vi "PWM_Lenkung.vi"(0 "vorne rechts":dbl=75.31181382488626, 1 "vorne links":dbl=29.917677039556622, 2 "Start":bool, 3 "Schräg links":dbl=31.586166184242515, 4 "Schräg rechts":dbl, 5 "PID Werte":T1={"proportional gain (Kc)"=0.5, "integral time (Ti, min)"=0.0, "derivative time (Td, min)"=0.002} {"proportional gain (Kc)" format="%#_10g"; "integral time (Ti, min)" format="%#_10g"; "derivative time (Td, min)" format="%#_10g"}) -> (14 "PWM Lenkung":dbl=0.3577035044911076)   [LabVIEW 2016]
doc: "PID Regelung für Servowert\n05.04.17_Tloe"
uses:
  <vilib>/addons/control/pid/pid.llb/PID (DBL).vi
  <vilib>/addons/control/pid/NI_PID_pid.lvlib
panel:
  in  "Abweichung (cm)":dbl=20.0 format="%#_13g"
  in  "Anteil Schräg":dbl=0.9
  # "vorher 0,9"
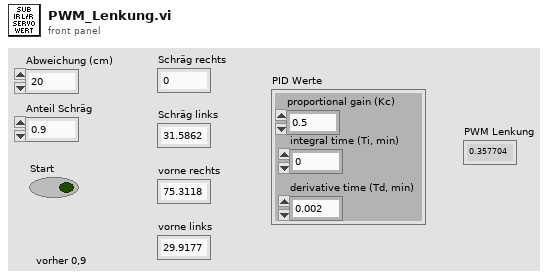
[diagram p1: front panel]
types:
  T1 = cluster{"proportional gain (Kc)":dbl, "integral time (Ti, min)":dbl, "derivative time (Td, min)":dbl}
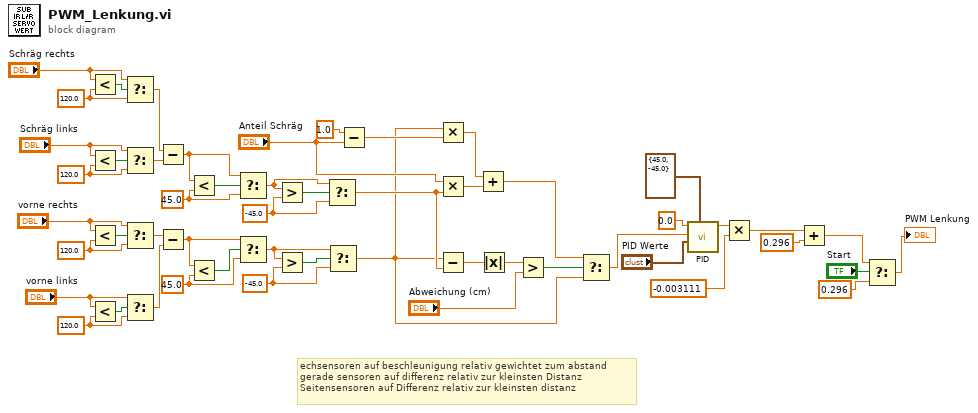
[diagram p0: block diagram]
diagram:
  w22 = 120.0 ("y")
  w26 = 120.0 ("y")
  w30 = 120.0 ("y")
  w33 = 120.0 ("y")
  w36 = -45.0 ("y")
  w39 = 45.0 ("y")
  w41 = -45.0 ("y")
  w44 = 45.0 ("y")
  # "echsensoren auf beschleunigung relativ gewichtet zum abstand\ngerade sensoren auf differenz relativ zur kleinsten Distanz\nSeitensensoren auf Differenz relativ zur kleinsten distanz"
  n1 = Less?(x="Schräg rechts", y=w26) -> (x < y?=w27:bool)
  n2 = Less?(x="Schräg links", y=w22) -> (x < y?=w23:bool)
  n3 = Less?(x="vorne rechts", y=w33) -> (x < y?=w35:bool)
  n4 = Less?(x="vorne links", y=w30) -> (x < y?=w31:bool)
  n5 = Select(t="Schräg rechts", s=w27, f=w26) -> (s? t:f=w25:dbl)
  n6 = Select(t="Schräg links", s=w23, f=w22) -> (s? t:f=w21:dbl)
  n7 = Select(t="vorne rechts", s=w35, f=w33) -> (s? t:f=w32:dbl)
  n8 = Select(t="vorne links", s=w31, f=w30) -> (s? t:f=w28:dbl)
  n9 = Subtract(x=w25, y=w21) -> (x-y=w9:dbl)
  n10 = Subtract(x=w32, y=w28) -> (x-y=w45:dbl)
  n11 = Less?(x=w9, y=w39) -> (x < y?=w40:bool)
  n12 = Less?(x=w45, y=w44) -> (x < y?=w46:bool)
  n13 = Select(t=w9, s=w40, f=w39) -> (s? t:f=w37:dbl)
  n14 = Select(t=w45, s=w46, f=w44) -> (s? t:f=w42:dbl)
  n15 = Greater?(x=w37, y=w36) -> (0:w38:bool)
  n16 = Greater?(x=w42, y=w41) -> (0:w43:bool)
  n17 = Select(t=w37, s=w38, f=w36) -> (s? t:f=w12:dbl)
  n18 = Select(t=w42, s=w43, f=w41) -> (s? t:f=w10:dbl)
  n19 = Subtract(x=1.0, y="Anteil Schräg") -> (x-y=w18:dbl)
  n20 = Multiply(x=w10, y=w18) -> (x*y=w19:dbl)
  n21 = Multiply(x="Anteil Schräg", y=w12) -> (x*y=w15:dbl)
  n22 = Subtract(x=w10, y=w12) -> (x-y=w7:dbl)
  n23 = Add(x=w19, y=w15) -> (x+y=w13:dbl)
  n24 = Absolute Value(x=w7) -> (abs(x)=w6:dbl)
  n25 = Greater?(x=w6, y="Abweichung (cm)") -> (0:w8:bool)
  n26 = Select(t=w13, s=w8, f=w10) -> (s? t:f=w5:dbl)
  n27 = call-poly <vilib>:"PID.vi"("output range"=cluster{"output high":dbl, "output low":dbl} {"output high"=45.0, "output low"=-45.0}, "PID gains"="PID Werte", "process variable"=w5, "setpoint"=0.0) -> ("output"=w52:dbl)  [unwired: 6 in, 1 out]
  n28 = Multiply(x=w52, y=-0.003111) -> (x*y=w49:dbl)
  n29 = Add(x=w49, y=0.296) -> (x+y=w4:dbl)
  n30 = Select(t=w4, s="Start", f=0.296) -> (s? t:f=→"PWM Lenkung":dbl)
